vi "Decode parameters.vi"(10 "Comminication in":T2(array[cluster]) {"ID" format="%.0x"; "DATA[0]" format="%.0x"; "DATA[1]" format="%.0x"; "DATA[2]" format="%.0x"; "DATA[3]" format="%.0x"; "DATA[4]" format="%.0x"; "DATA[5]" format="%.0x"; "DATA[6]" format="%.0x"; "DATA[7]" format="%.0x"}, 11 "Commands":T1) -> (2 "Numeric results":sgl[](array[numeric]) format="%#_13g", 3 "String results":string)   [LabVIEW 2025]
uses:
  Commands.ctl
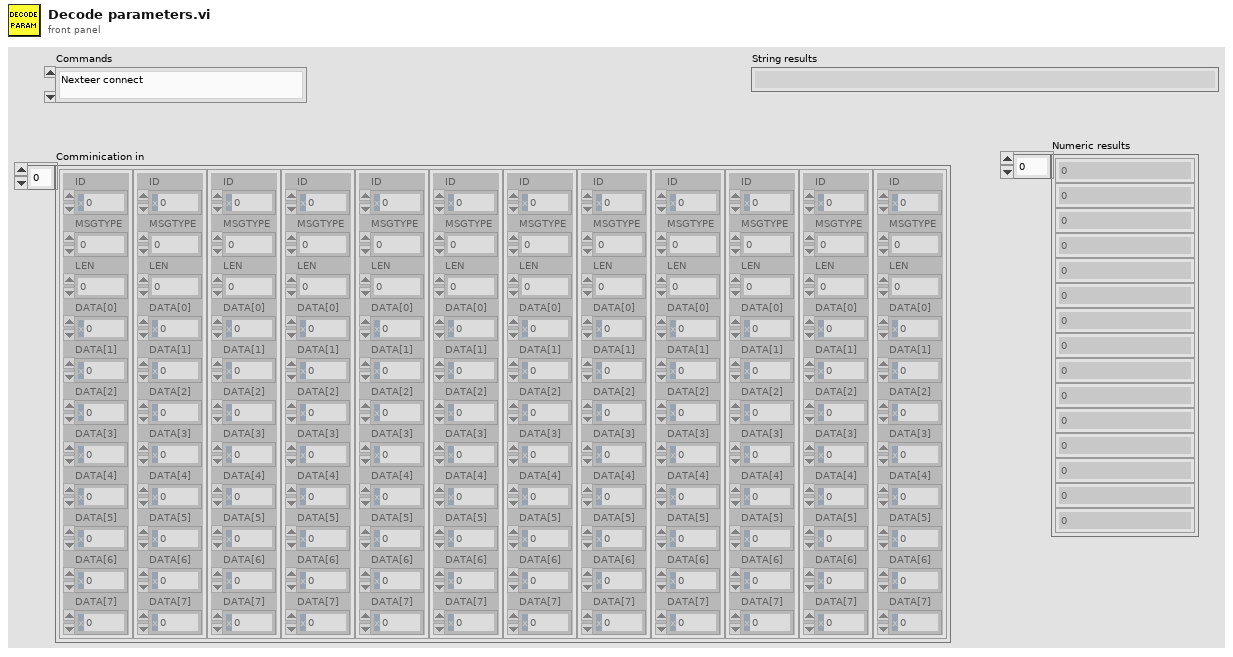
[diagram p1: front panel]
types:
  T1 = typedef "Commands.ctl" = enum16{"Nexteer connect", "Write Polarity", "Write BEMF", "Write Torque Scale Sensors T1", "Write Torque Scale Sensors T2", "Trim HW Torque Sensors T1", "Trim HW Torque Sensors T2", "Read HW Torque Trim Performed Sensors T1", "Read HW Torque Trim Performed Sensors T2", "Write EOL Offset values to defaults", "Write EOL Gain values to defaults", "Write Serial Number", "Write Hardware Part Number", "Write EPS Serial Number", "Read MEC Counter", "MCU Reset", "Read System State", "Read First Motor Position", "Manufacturing Diagnostic Defeat", "Perform Current Offset ", "Current Offset Status", "Enable Engine Run", "Perform Current Gain ", "Current Gain Status", "Disable Torque Ramp Down ", "Disable Engine Run", "Set Vehicle Speed Override", "Read Offset Values Using FD F5", "Read Gain Values Using FD F4", "Clear Nexteer NTCs", "Read Second Motor Position", "Read ECU Software ID", "Read Internal Software Version", "Read Bootloader ID", "Read Bootloader Software Version", "Read Calibration Release 0", "Read Calibration Release 1", "Read Calibration Release 2", "Read Temperature  ", "Battery Voltage  ", "Read Motor Angle 0", "Read Motor Angle 1 ", "Set Motor Torque Command ", "Read Motor Current   ", "Stop Motor Torque Command", "Read NTCs", "Read Serial Number", "Read HW Part Number", "Read Polarity", "Set NVM Access Defeat", "Read Software Release", "Read Software Build Date", "Write Single Inverter Hardware value", "Write Dual Inverter Hardware value", "Read Single Inverter HW Value", "Read Dual Inverter HW Value", "Write MEC Counter FE", "Write MEC Counter FF", "Read BEMF", "Read Torque 1 FDB6", "Read Torque 2 FDB7", "Read Torque Trim 1 FDB4", "Read Torque Trim 2 FDB5", "Write Torque Trim 1 FDB4", "Write Torque Trim 2 FDB5", "XCP connect", "Read HW Torque T1", "Read HW Torque T2", "Read Motor Speed "}
  T2 = cluster{"ID":u32, "MSGTYPE":u8, "LEN":u8, "DATA[0]":u8, "DATA[1]":u8, "DATA[2]":u8, "DATA[3]":u8, "DATA[4]":u8, "DATA[5]":u8, "DATA[6]":u8, "DATA[7]":u8}[]
  T3 = cluster{"ID":u32, "MSGTYPE":u8, "LEN":u8, "DATA[0]":u8, "DATA[1]":u8, "DATA[2]":u8, "DATA[3]":u8, "DATA[4]":u8, "DATA[5]":u8, "DATA[6]":u8, "DATA[7]":u8}
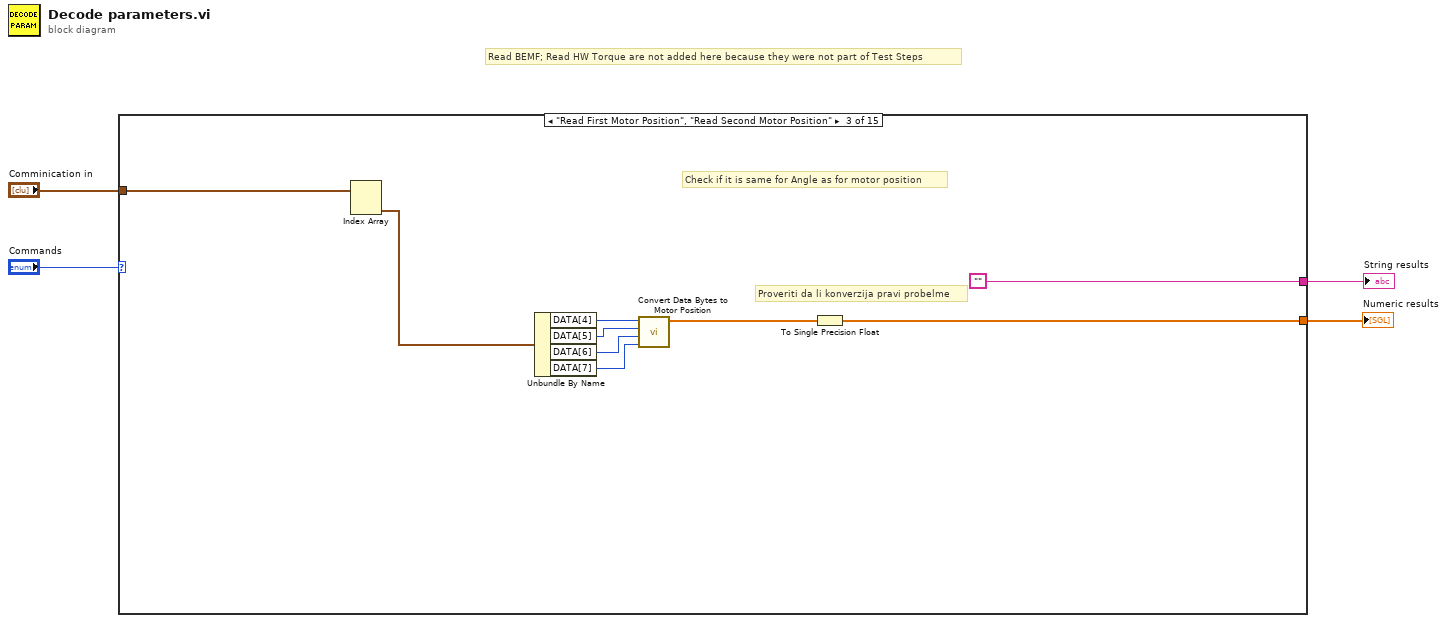
[diagram p0: block diagram]
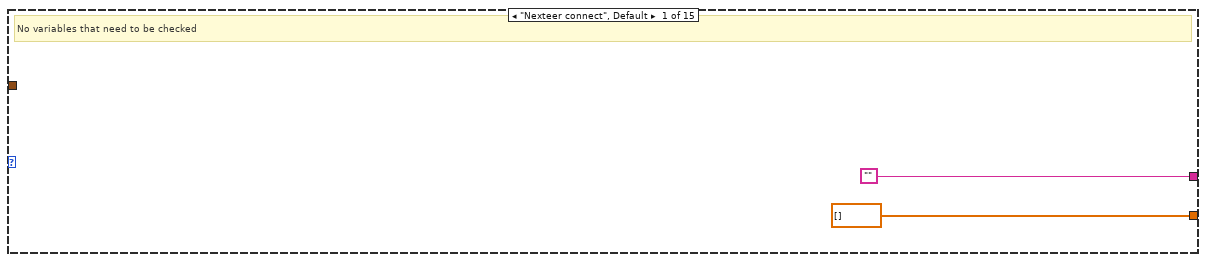
[diagram p2: hidden frame]
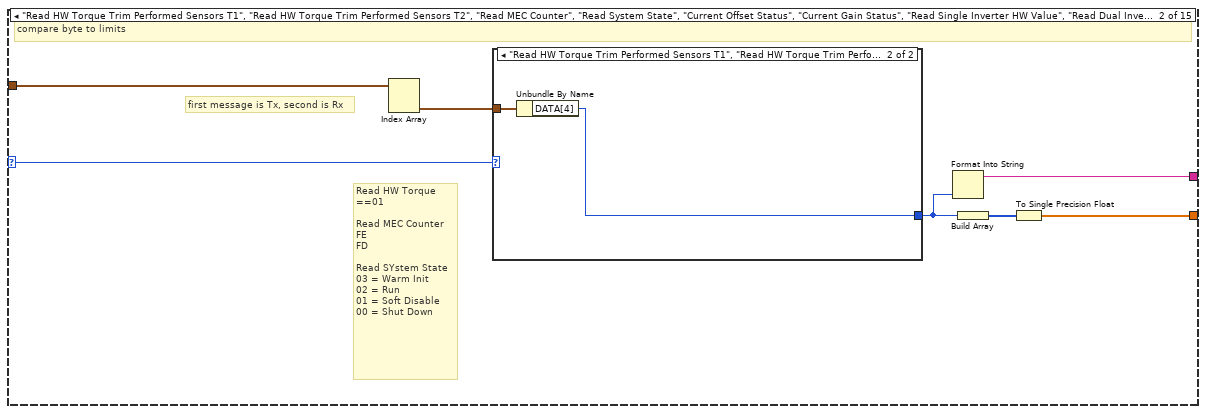
[diagram p3: hidden frame]
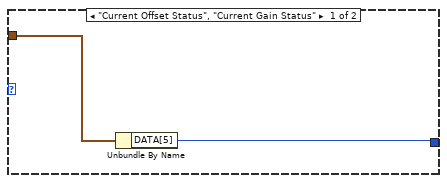
[diagram p4: hidden frame]
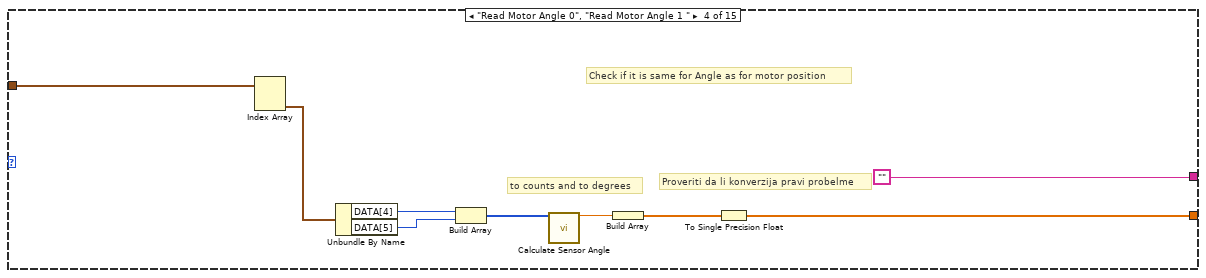
[diagram p5: hidden frame]
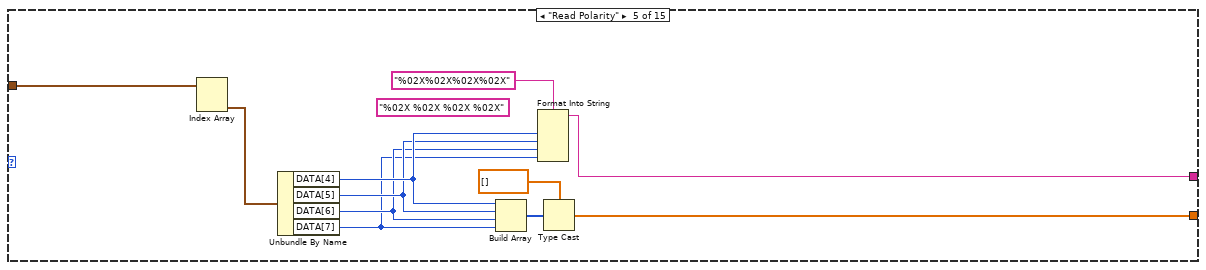
[diagram p6: hidden frame]
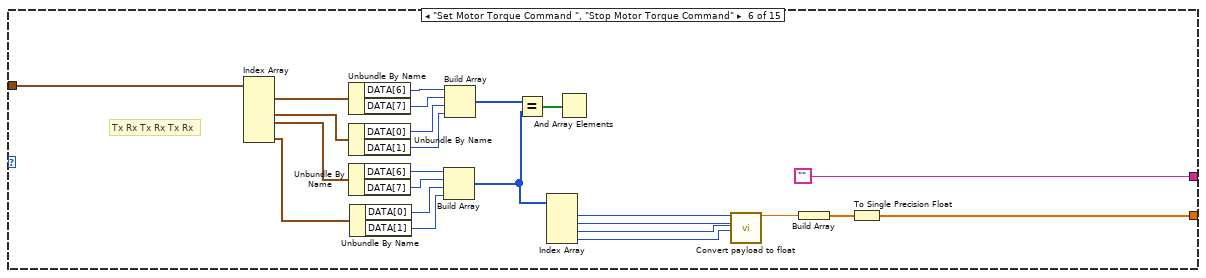
[diagram p7: hidden frame]
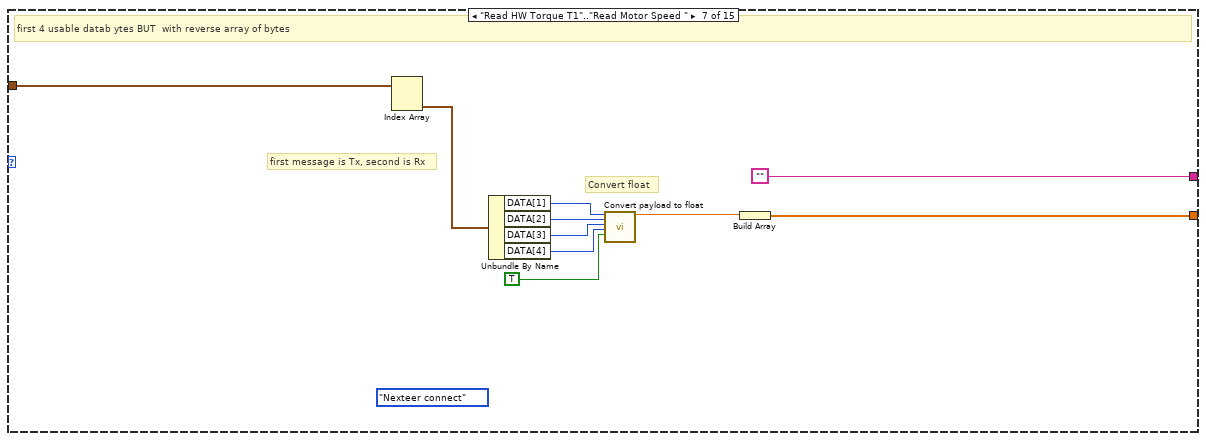
[diagram p8: hidden frame]
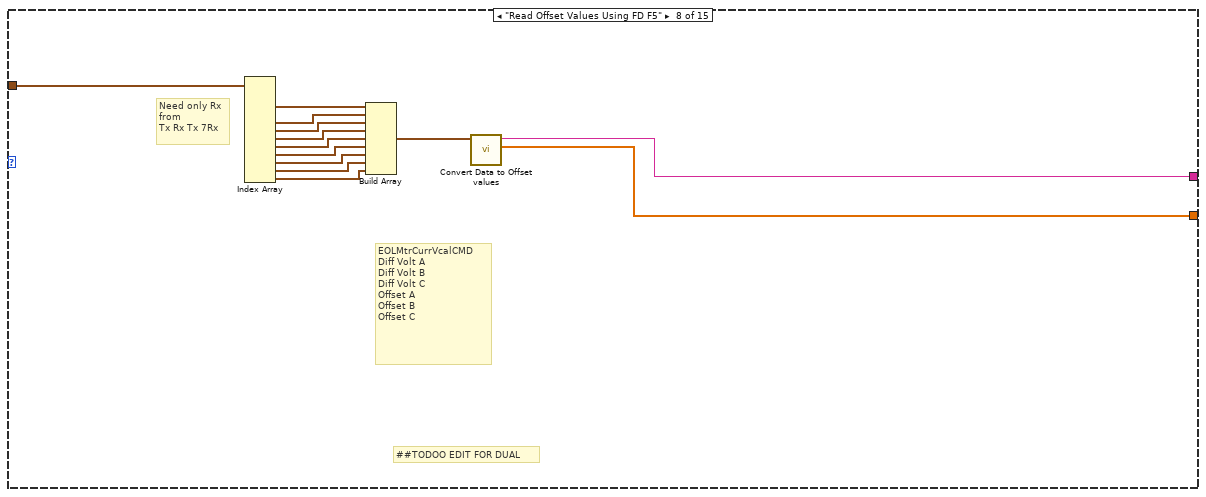
[diagram p9: hidden frame]
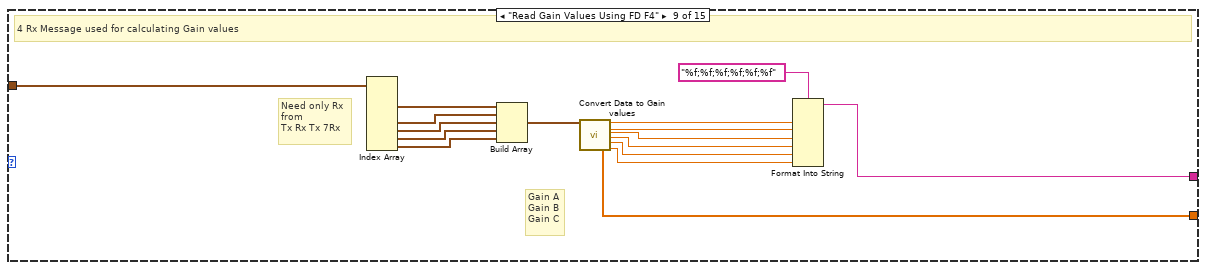
[diagram p10: hidden frame]
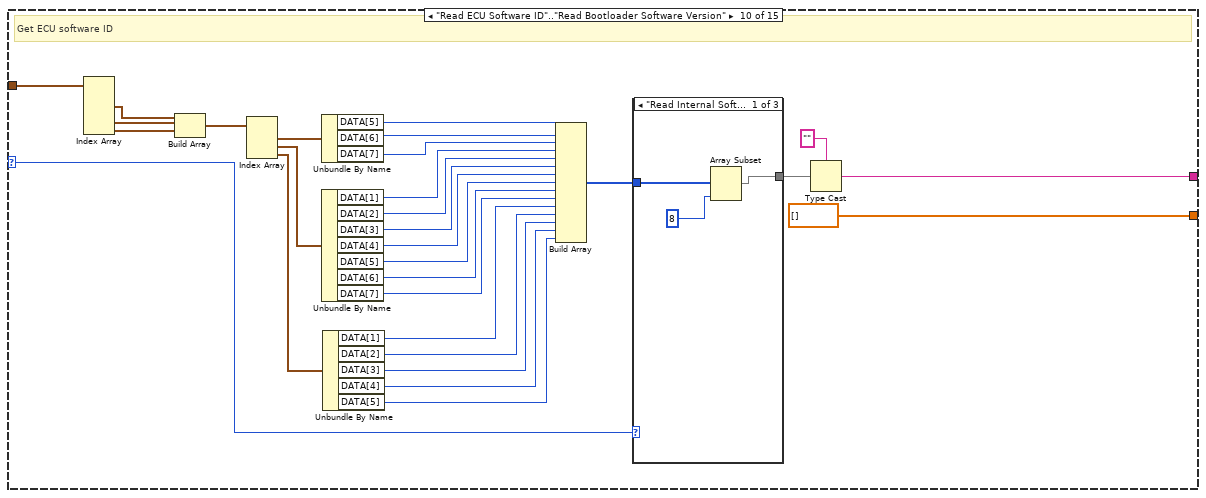
[diagram p11: hidden frame]
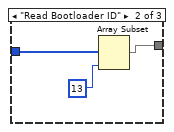
[diagram p12: hidden frame]
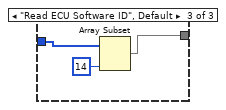
[diagram p13: hidden frame]
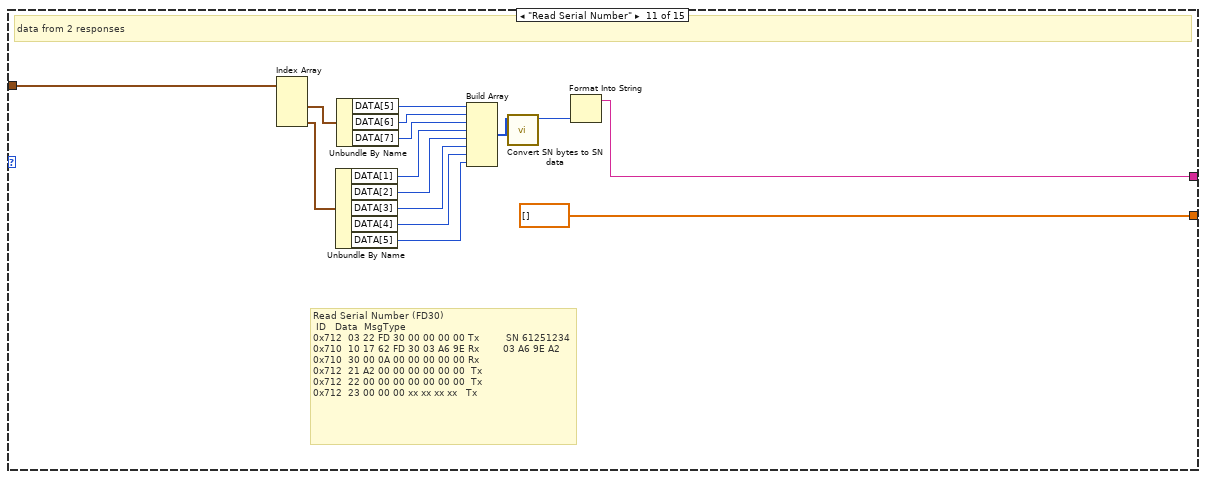
[diagram p14: hidden frame]
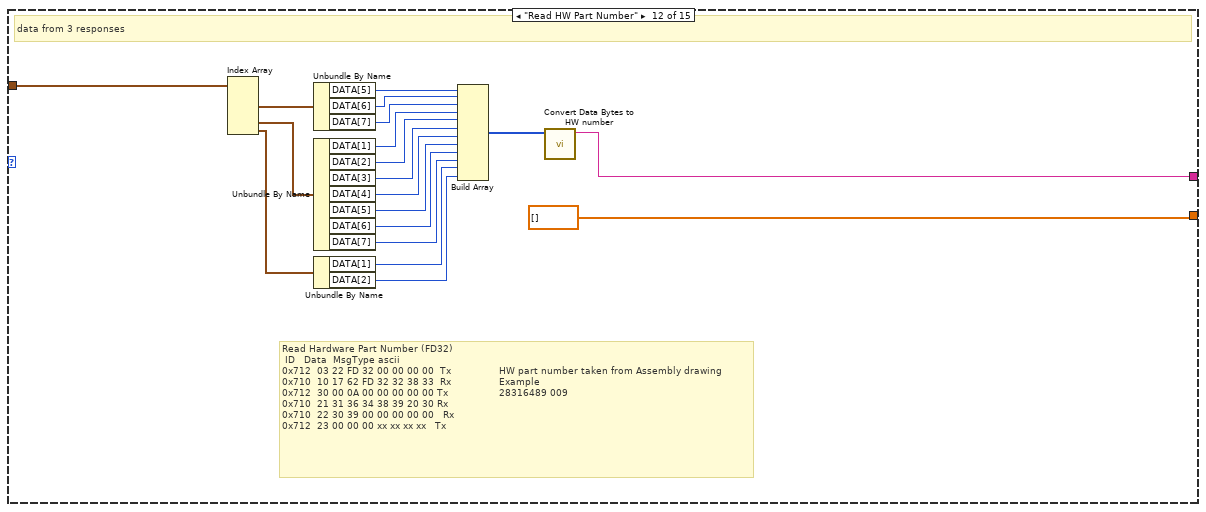
[diagram p15: hidden frame]
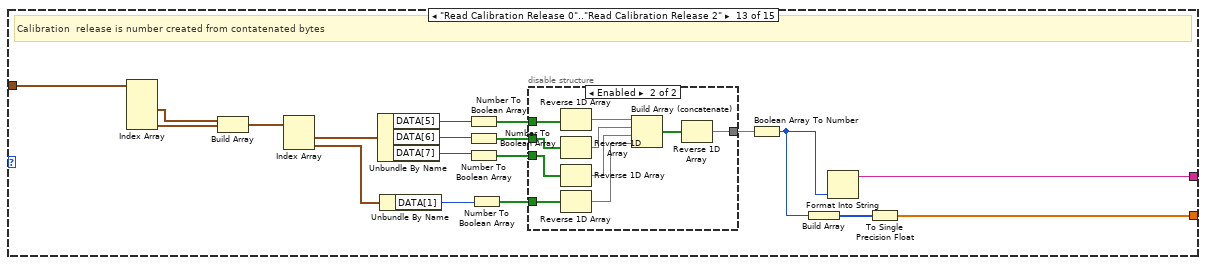
[diagram p16: hidden frame]
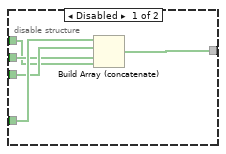
[diagram p17: hidden frame]
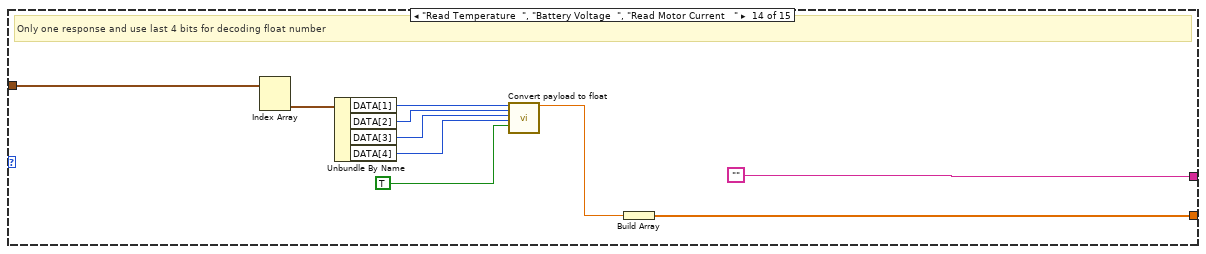
[diagram p18: hidden frame]
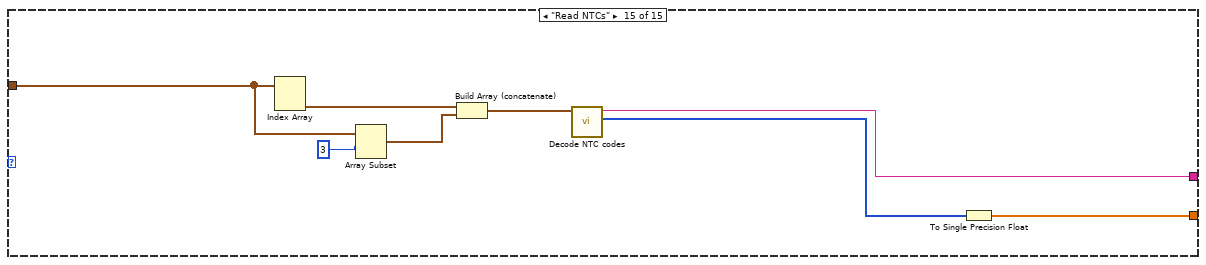
[diagram p19: hidden frame]
diagram:
  # "Read BEMF; Read HW Torque are not added here because they were not part of Test Steps"
  n1 = case shown="\"Read First Motor Position\", \"Read Second Motor Position\"" "Commands" {
    selector: "Commands" -> [_ w10 _ _ _ _ _ _ _ w113 _ _ _ _ _]
    tunnel: "Comminication in" -> [_ w13 w26 w29 w45 w70 w80 w93 w104 w138 w162 w175 w197 w225 w233]
    tunnel: ["" w7 "" "" w37 "" "" w82 w95 w111 w153 w165 w182 "" w228] -> w2
    tunnel: [sgl[] [] ("Numeric results") w9 w18 w28 w43 w47 w78 w81 w94 sgl[] [] ("Numeric results") sgl[] [] ("Numeric results") sgl[] [] ("Numeric results") w184 w217 w226] -> w1
    frame "Nexteer connect", Default {
      # "No variables that need to be checked"
    }
    frame "Read HW Torque Trim Performed Sensors T1", "Read HW Torque Trim Performed Sensors T2", "Read MEC Counter", "Read System State", "Current Offset Status", "Current Gain Status", "Read Single Inverter HW Value", "Read Dual Inverter HW Value" {
      # "Read HW Torque\n==01\n\nRead MEC Counter\nFE\nFD\n\nRead SYstem State\n03\t=\tWarm Init\n02\t=\tRun\n01\t=\tSoft Disable\n00\t=\tShut Down"
      # "first message is Tx, second is Rx"
      # "compare byte to limits"
      n2 = Index Array(array=w13) -> (element #2=w12:T3)  [unwired: 2 in, 1 out]
      n3 = case shown="\"Read HW Torque Trim Performed Sensors T1\", \"Read HW Torque Trim Performed Sensors T2\", \"Read MEC Counter\", \"Read System State\", \"Read Single Inverter HW Value\", \"Read Dual Inverter HW Value\", Default" w10 {
        tunnel: w12 -> [w15 w17]
        tunnel: [w14 w16] -> w8
        frame "Current Offset Status", "Current Gain Status" {
          n4 = Unbundle By Name(w15) -> ("DATA[5]"=w14:u8)
        }
        frame "Read HW Torque Trim Performed Sensors T1", "Read HW Torque Trim Performed Sensors T2", "Read MEC Counter", "Read System State", "Read Single Inverter HW Value", "Read Dual Inverter HW Value", Default {
          n5 = Unbundle By Name(w17) -> ("DATA[4]"=w16:u8)
        }
      }
      n6 = Format Into String(w8) -> (resulting string=w7:string)  [unwired: 3 in, 1 out]
      n7 = Build Array(w8) -> (w11:u8[])
      n8 = To Single Precision Float(number=w11) -> (single precision float=w9:sgl[])
    }
    frame "Read First Motor Position", "Read Second Motor Position" {
      # "Proveriti da li konverzija pravi probelme"
      # "Check if it is same for Angle as for motor position"
      n9 = Index Array(array=w26) -> (element #2=w25:T3)  [unwired: 2 in, 1 out]
      n10 = Unbundle By Name(w25) -> ("DATA[4]"=w23:u8, "DATA[5]"=w22:u8, "DATA[6]"=w21:u8, "DATA[7]"=w20:u8)
      n11 = call "Convert Data Bytes to Motor Position.vi"("DATA[7]"=w20, "DATA[6]"=w21, "DATA[5]"=w22, "DATA[4]"=w23) -> ("Motor Position"=w19:sgl[])  [unwired: 7 in]
      n12 = To Single Precision Float(number=w19) -> (single precision float=w18:sgl[])
    }
    frame "Read Motor Angle 0", "Read Motor Angle 1 " {
      # "Proveriti da li konverzija pravi probelme"
      # "Check if it is same for Angle as for motor position"
      # "to counts and to degrees"
      n13 = Index Array(array=w29) -> (element #2=w35:T3)  [unwired: 2 in, 1 out]
      n14 = Unbundle By Name(w35) -> ("DATA[4]"=w34:u8, "DATA[5]"=w33:u8)
      n15 = Build Array(w34, w33) -> (w32:u8[])
      n16 = call "Calculate Sensor Angle.vi"("DATA[4-5]"=w32) -> ("Degree0"=w31:dbl)  [unwired: 17 in, 1 out]
      n17 = Build Array(w31) -> (w30:dbl[])
      n18 = To Single Precision Float(number=w30) -> (single precision float=w28:sgl[])
    }
    frame "Read Polarity" {
      (unwired) "%02X %02X %02X %02X" ("format string")
      n19 = Index Array(array=w45) -> (element #2=w46:T3)  [unwired: 2 in, 1 out]
      n20 = Unbundle By Name(w46) -> ("DATA[4]"=w41:u8, "DATA[5]"=w40:u8, "DATA[6]"=w39:u8, "DATA[7]"=w38:u8)
      n21 = Build Array(w41, w40, w39, w38) -> (w42:u8[])
      n22 = Format Into String(format string="%02X%02X%02X%02X", w41, w40, w39, w38) -> (resulting string=w37:string)  [unwired: 2 in, 1 out]
      n23 = Type Cast(type=sgl[] [] ("Numeric results"), x=w42) -> (*(type *) &x=w43:sgl[])
    }
    frame "Set Motor Torque Command ", "Stop Motor Torque Command" {
      # "Tx Rx Tx Rx Tx Rx"
      n24 = Index Array(array=w70) -> (element #1=w69:T3, element #3=w68:T3, element #4=w67:T3, element #6=w66:T3)  [unwired: 6 in, 2 out]
      n25 = Unbundle By Name(w69) -> ("DATA[6]"=w65:u8, "DATA[7]"=w64:u8)
      n26 = Unbundle By Name(w68) -> ("DATA[0]"=w63:u8, "DATA[1]"=w62:u8)
      n27 = Unbundle By Name(w67) -> ("DATA[6]"=w61:u8, "DATA[7]"=w60:u8)
      n28 = Unbundle By Name(w66) -> ("DATA[0]"=w59:u8, "DATA[1]"=w58:u8)
      n29 = Build Array(w61, w60, w59, w58) -> (w55:u8[])
      n30 = Build Array(w65, w64, w63, w62) -> (w57:u8[])
      n31 = Equal?(x=w57, y=w55) -> (x = y?=w56:bool[])
      n32 = Index Array(array=w55) -> (element #1=w54:u8, element #2=w53:u8, element #3=w52:u8, element #4=w51:u8)  [unwired: 4 in]
      n33 = And Array Elements(Boolean array=w56) -> ()  [unwired: 1 out]
      n34 = call "Convert payload to float.vi"("Byte1"=w54, "Byte2"=w53, "Byte3"=w52, "Byte4"=w51) -> ("FloatNumber"=w50:sgl)  [unwired: 15 in]
      n35 = Build Array(w50) -> (w49:sgl[])
      n36 = To Single Precision Float(number=w49) -> (single precision float=w47:sgl[])
    }
    frame "Read HW Torque T1".."Read Motor Speed " {
      (unwired) Commands."Nexteer connect" ("Commands 2")
      # "Convert float"
      # "first message is Tx, second is Rx"
      # "first 4 usable datab ytes BUT  with reverse array of bytes"
      n37 = Index Array(array=w80) -> (element #2=w79:T3)  [unwired: 2 in, 1 out]
      n38 = Unbundle By Name(w79) -> ("DATA[1]"=w77:u8, "DATA[2]"=w76:u8, "DATA[3]"=w75:u8, "DATA[4]"=w74:u8)
      n39 = call "Convert payload to float.vi"("Byte1"=w77, "Byte2"=w76, "Byte3"=w75, "Byte4"=w74, "Invert"=TRUE) -> ("FloatNumber"=w72:sgl)  [unwired: 14 in]
      n40 = Build Array(w72) -> (w78:sgl[])
    }
    frame "Read Offset Values Using FD F5" {
      # "##TODOO EDIT FOR DUAL"
      # "EOLMtrCurrVcalCMD\nDiff Volt A\nDiff Volt B\nDiff Volt C\nOffset A\nOffset B\nOffset C"
      # "Need only Rx\nfrom\nTx Rx Tx 7Rx"
      n41 = Index Array(array=w93) -> (element #2=w92:T3, element #4=w91:T3, element #5=w90:T3, element #6=w89:T3, element #7=w88:T3, element #8=w86:T3, element #9=w85:T3, element #10=w84:T3, element #11=w83:T3)  [unwired: 11 in, 2 out]
      n42 = Build Array(w92, w91, w90, w89, w88, w86, w85, w84, w83) -> (w87:T2)
      n43 = call "Convert Data to Offset values.vi"("Messages"=w87) -> ("all values"=w81:sgl[], "Values"=w82:string)  [unwired: 9 in]
    }
    frame "Read Gain Values Using FD F4" {
      # "Gain A\nGain B\nGain C"
      # "Need only Rx\nfrom\nTx Rx Tx 7Rx"
      # "4 Rx Message used for calculating Gain values"
      n44 = Index Array(array=w104) -> (element #2=w109:T3, element #4=w108:T3, element #5=w107:T3, element #6=w106:T3, element #7=w105:T3)  [unwired: 7 in, 2 out]
      n45 = Build Array(w109, w108, w107, w106, w105) -> (w103:T2)
      n46 = call "Convert Data to Gain values.vi"("Messages"=w103) -> ("Gain values"=w94:sgl[], "Gain A"=w102:sgl, "Gain B"=w101:sgl, "Gain C"=w100:sgl, "Gain D"=w99:sgl, "Gain E"=w98:sgl, "Gain F"=w97:sgl)  [unwired: 12 in]
      n47 = Format Into String(format string="%f;%f;%f;%f;%f;%f", w102, w101, w100, w99, w98, w97) -> (resulting string=w95:string)  [unwired: 2 in, 1 out]
    }
    frame "Read ECU Software ID".."Read Bootloader Software Version" {
      # "Get ECU software ID"
      n48 = Index Array(array=w138) -> (element #2=w137:T3, element #4=w136:T3, element #5=w135:T3)  [unwired: 5 in, 2 out]
      n49 = Build Array(w137, w136, w135) -> (w134:T2)
      n50 = Index Array(array=w134) -> (element #1=w133:T3, element #2=w132:T3, element #3=w131:T3)  [unwired: 3 in]
      n51 = Unbundle By Name(w133) -> ("DATA[5]"=w130:u8, "DATA[6]"=w129:u8, "DATA[7]"=w128:u8)
      n52 = Unbundle By Name(w132) -> ("DATA[1]"=w127:u8, "DATA[2]"=w126:u8, "DATA[3]"=w125:u8, "DATA[4]"=w124:u8, "DATA[5]"=w123:u8, "DATA[6]"=w122:u8, "DATA[7]"=w121:u8)
      n53 = Unbundle By Name(w131) -> ("DATA[1]"=w120:u8, "DATA[2]"=w119:u8, "DATA[3]"=w118:u8, "DATA[4]"=w117:u8, "DATA[5]"=w116:u8)
      n54 = Build Array(w130, w129, w128, w127, w126, w125, w124, w123, w122, w121, w120, w119, w118, w117, w116) -> (w114:u8[])
      n55 = case shown="\"Read Internal Software Version\", \"Read Bootloader Software Version\"" w113 {
        tunnel: w114 -> [w141 w143 w147]
        tunnel: [w139 w142 w146] -> w110
        frame "Read Internal Software Version", "Read Bootloader Software Version" {
          n56 = Array Subset(array=w141, length=8) -> (w139:u8[])  [unwired: 1 in]
        }
        frame "Read Bootloader ID" {
          n57 = Array Subset(array=w143, length=13) -> (w142:u8[])  [unwired: 1 in]
        }
        frame "Read ECU Software ID", Default {
          n58 = Array Subset(array=w147, length=14) -> (w146:u8[])  [unwired: 1 in]
        }
      }
      n59 = Type Cast(type="", x=w110) -> (*(type *) &x=w111:string)
    }
    frame "Read Serial Number" {
      # "Read Serial Number (FD30)\t\t\t\t\n ID\t\t Data\t MsgType\t\n0x712\t\t03 22 FD 30 00 00 00 00\tTx        \tSN 61251234\n0x710\t\t10 17 62 FD 30 03 A6 9E\tRx        03 A6 9E A2\n0x710\t\t30 00 0A 00 00 00 00 00\tRx\t\n0x712\t\t21 A2 00 00 00 00 00 00 \tTx\t\n0x712\t\t22 00 00 00 00 00 00 00 \tTx\t\n0x712\t\t23 00 00 00 xx xx xx xx  \tTx"
      # "data from 2 responses"
      n60 = Index Array(array=w162) -> (element #2=w161:T3, element #4=w160:T3)  [unwired: 4 in, 2 out]
      n61 = Unbundle By Name(w160) -> ("DATA[1]"=w156:u8, "DATA[2]"=w151:u8, "DATA[3]"=w150:u8, "DATA[4]"=w149:u8, "DATA[5]"=w148:u8)
      n62 = Unbundle By Name(w161) -> ("DATA[5]"=w159:u8, "DATA[6]"=w158:u8, "DATA[7]"=w157:u8)
      n63 = Build Array(w159, w158, w157, w156, w151, w150, w149, w148) -> (w155:u8[])
      n64 = call "Convert SN bytes to SN data.vi"("SN Data Bytes"=w155) -> ("SN"=w154:u32)  [unwired: 9 in, 1 out]
      n65 = Format Into String(w154) -> (resulting string=w153:string)  [unwired: 3 in, 1 out]
    }
    frame "Read HW Part Number" {
      # "Read Hardware Part Number (FD32)\t\t\t\t\n ID\t\t Data\t MsgType\tascii\n0x712\t\t03 22 FD 32 00 00 00 00 \tTx\t               HW part number taken from Assembly drawing\n0x710\t\t10 17 62 FD 32 32 38 33 \tRx\t               Example\n0x712\t\t30 00 0A 00 00 00 00 00\tTx\t                28316489 009 \n0x710\t\t21 31 36 34 38 39 20 30\tRx\t\n0x710\t\t22 30 39 00 00 00 00 00  \tRx\t\n0x712\t\t23 00 00 00 xx xx xx xx  \tTx"
      # "data from 3 responses"
      n66 = Index Array(array=w175) -> (element #2=w181:T3, element #4=w180:T3, element #5=w163:T3)  [unwired: 5 in, 2 out]
      n67 = Unbundle By Name(w181) -> ("DATA[5]"=w179:u8, "DATA[6]"=w178:u8, "DATA[7]"=w177:u8)
      n68 = Unbundle By Name(w180) -> ("DATA[1]"=w176:u8, "DATA[2]"=w174:u8, "DATA[3]"=w173:u8, "DATA[4]"=w172:u8, "DATA[5]"=w171:u8, "DATA[6]"=w170:u8, "DATA[7]"=w169:u8)
      n69 = Unbundle By Name(w163) -> ("DATA[1]"=w168:u8, "DATA[2]"=w167:u8)
      n70 = Build Array(w179, w178, w177, w176, w174, w173, w172, w171, w170, w169, w168, w167) -> (w166:u8[])
      n71 = call "Convert Data Bytes to HW number.vi"("Bytes"=w166) -> ("HW part number"=w165:string)  [unwired: 10 in]
    }
    frame "Read Calibration Release 0".."Read Calibration Release 2" {
      # "Calibration  release is number created from contatenated bytes"
      n72 = Index Array(array=w197) -> (element #2=w200:T3, element #4=w199:T3)  [unwired: 4 in, 2 out]
      n73 = Build Array(w200, w199) -> (w198:T2)
      n74 = Index Array(array=w198) -> (element #1=w196:T3, element #2=w195:T3)  [unwired: 2 in]
      n75 = Unbundle By Name(w196) -> ("DATA[5]"=w191:u8, "DATA[6]"=w192:u8, "DATA[7]"=w193:u8)
      n76 = Unbundle By Name(w195) -> ("DATA[1]"=w194:u8)
      n77 = Number To Boolean Array(number=w191) -> (Boolean array=w186:bool[])
      n78 = Number To Boolean Array(number=w192) -> (Boolean array=w187:bool[])
      n79 = Number To Boolean Array(number=w193) -> (Boolean array=w188:bool[])
      n80 = Number To Boolean Array(number=w194) -> (Boolean array=w189:bool[])
      n81 = disable-structure shown="Enabled" {
        disable-tunnel: w189 -> [w205 w212]
        disable-tunnel: w188 -> [w204 w213]
        disable-tunnel: w187 -> [w203 w214]
        disable-tunnel: w186 -> [w202 w215]
        disable-tunnel: [w201 w206] -> w185
        frame Disabled {
          n82 = Build Array (concatenate)(w205, w204, w203, w202) -> (w201:bool[])
        }
        frame Enabled {
          n83 = Reverse 1D Array(array=w215) -> (reversed array=w211:bool[])
          n84 = Reverse 1D Array(array=w214) -> (reversed array=w210:bool[])
          n85 = Reverse 1D Array(array=w213) -> (reversed array=w209:bool[])
          n86 = Reverse 1D Array(array=w212) -> (reversed array=w208:bool[])
          n87 = Build Array (concatenate)(w211, w210, w209, w208) -> (w207:bool[])
          n88 = Reverse 1D Array(array=w207) -> (reversed array=w206:bool[])
        }
      }
      n89 = Boolean Array To Number(Boolean array=w185) -> (number=w183:u32)
      n90 = Build Array(w183) -> (w190:u32[])
      n91 = Format Into String(w183) -> (resulting string=w182:string)  [unwired: 3 in, 1 out]
      n92 = To Single Precision Float(number=w190) -> (single precision float=w184:sgl[])
    }
    frame "Read Temperature  ", "Battery Voltage  ", "Read Motor Current   " {
      # "Only one response and use last 4 bits for decoding float number"
      n93 = Index Array(array=w225) -> (element #2=w224:T3)  [unwired: 2 in, 1 out]
      n94 = Unbundle By Name(w224) -> ("DATA[1]"=w223:u8, "DATA[2]"=w222:u8, "DATA[3]"=w221:u8, "DATA[4]"=w220:u8)
      n95 = call "Convert payload to float.vi"("Byte1"=w223, "Byte2"=w222, "Byte3"=w221, "Byte4"=w220, "Invert"=TRUE) -> ("FloatNumber"=w218:sgl)  [unwired: 14 in]
      n96 = Build Array(w218) -> (w217:sgl[])
    }
    frame "Read NTCs" {
      n97 = Index Array(array=w233) -> (element #2=w231:T3)  [unwired: 2 in, 1 out]
      n98 = Array Subset(array=w233, index=3) -> (w230:T2)  [unwired: 1 in]
      n99 = Build Array (concatenate)(w231, w230) -> (w229:T2)
      n100 = call "Decode NTC codes.vi"("NTC Messages"=w229) -> ("NTC codes"=w227:u32[], "NTCs"=w228:string)  [unwired: 9 in]
      n101 = To Single Precision Float(number=w227) -> (single precision float=w226:sgl[])
    }
  }
  "String results" <- w2
  "Numeric results" <- w1
